vi "AddChecksum.vi"(2 "String IN":string) -> (7 "OUT":string)   [LabVIEW 2014]
doc: "Add checksum to string"
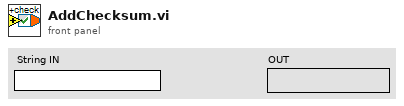
[diagram p1: front panel]
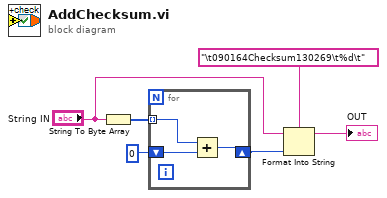
[diagram p0: block diagram]
diagram:
  n1 = String To Byte Array(string="String IN") -> (unsigned byte array=w6:u8[])
  n2 = for {
    tunnel: w6 -> [w8] mode=indexing
    shift-right: [w7] -> w4
    shift-left: u64 0 -> [w9]
    n3 = Add(x=w8, y=w9) -> (x+y=w7:u64)
  }
  n4 = Format Into String(format string="\t090164Checksum130269\t%d\t", initial string="String IN", w4) -> (resulting string=→"OUT":string)  [unwired: 1 in, 1 out]
